vi "Read Time Stamp.vi"(11 "Properties in":refnum<class "Properties.lvclass">) -> (2 "Time Stamp":timestamp, 3 "Properties out":refnum<class "Properties.lvclass">)   [LabVIEW 2020, in "Caraya.lvlib" / "Properties.lvclass"]
uses:
  Properties.lvclass
  Properties.lvclass/Properties.ctl
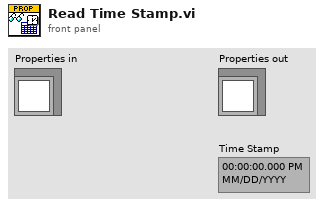
[diagram p1: front panel]
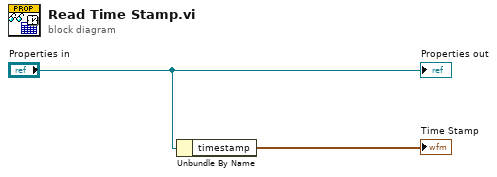
[diagram p0: block diagram]
diagram:
  n1 = Unbundle By Name("Properties in") -> ("timestamp"=→"Time Stamp":timestamp)
  "Properties out" <- "Properties in"
